vi "Lesson5 - auto-indexing.vi"() -> ()   [LabVIEW 2013]
panel:
  out "Array 2":i32[](array[numeric])
  out "Array":dbl[](array[numeric]) format="%.2f"
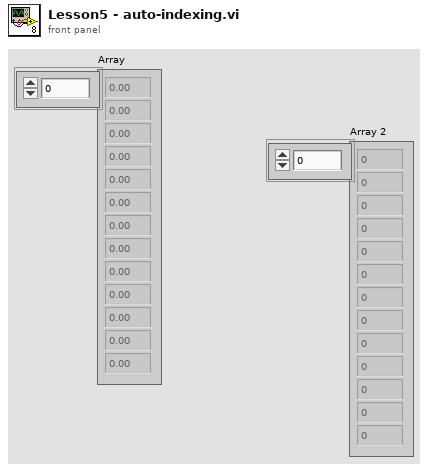
[diagram p1: front panel]
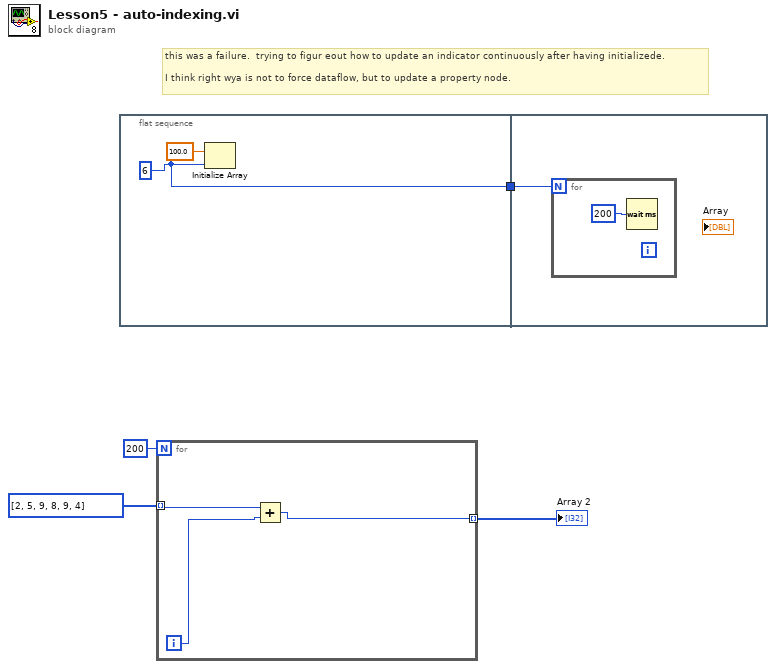
[diagram p0: block diagram]
diagram:
  # "this was a failure.  trying to figur eout how to update an indicator continuously after having initializede.\n\nI think right wya is not to force dataflow, but to update a property node."
  n1 = flat-sequence {
    tunnel: [w5] -> w4
    tunnel: w4 -> [w7]
    frame #0 {
      w5 = 6
      n2 = Initialize Array(100.0 ("element"), w5) -> ()  [unwired: 1 out]
    }
    frame #1 {
      n3 = for {
        N: w7 -> [_]
        n4 = Wait (ms)(milliseconds to wait=u32 200) -> ()  [unwired: 1 out]
      }
    }
  }
  n5 = for {
    N: 200 -> [_]
    tunnel: i32[] [2, 5, 9, 8, 9, 4] -> [w10] mode=indexing
    tunnel: [w11] -> w1 mode=indexing
    i -> [w9]
    n6 = Add(x=w10, y=w9) -> (x+y=w11:i32)
  }
  "Array 2" <- w1
